vi "BRig_dataExp_Audio_amp_L.vi"() -> (2 "output_Audio_amp__L":i32)   [LabVIEW 2014]
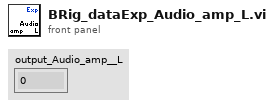
[diagram p1: front panel]
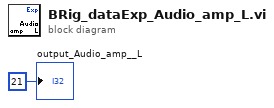
[diagram p0: block diagram]
diagram:
  "output_Audio_amp__L" <- 21 ("output_iBlock")
